vi "SerialCom Initialize.vi"(8 "error in (no error)":errorcluster) -> (0 "error out":errorcluster, 3 "VISA resource name out":refnum<visa-resource-name>)   [LabVIEW 2022 SP3]
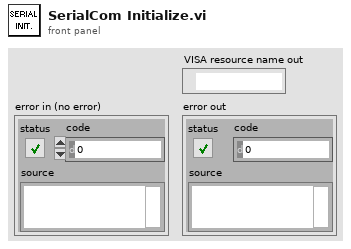
[diagram p1: front panel]
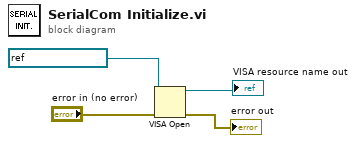
[diagram p0: block diagram]
diagram:
  n1 = VISA Open(error in (no error)="error in (no error)", VISA resource name=refnum<visa-resource-name> "ControlBoard" ("ControlBoard VISA")) -> (VISA resource name=→"VISA resource name out":refnum<visa-resource-name>, error out=→"error out":errorcluster)  [unwired: 3 in]
